vi "ReadScheduleFile.vi"(7 "Enum":enum16{"Load", "Get"}(ring), 8 "Team Info / Schedule File":path=path "C:/Program Files/FIRST LEGO LEAGUE TOURNAMENT/data/schedule.csv") -> (0 "error out":errorcluster, 1 "Table Stats":T1, 2 "PracticeMatches":string[][](array[string])=[["1", "1060", "3132", "5421", "77"], ["2", "510", "2128", "5441", "781"], ["3", "305", "98", "5470", "1951"], ["4", "685", "1429", "5481", "340"], ["5", "486", "3730", "5420", "12"], ["6", "1857", "3019", "5411", "390"], ["7", "5391", "1105", "5400", "2580"], ["8", "729", "2216", "5480", "822"], ["9", "752", "266", "5371", "3187"], ["10", "3622", "4861", "5360", "517"], ["11", "1633", "2882", "0", "0"], ["12", "3132", "5421", "77", "1060"], ["13", "2128", "5441", "781", "510"], ["14", "98", "5470", "1951", "305"], ["15", "1429", "5481", "340", "685"], ["16", "3730", "5420", "12", "486"], ["17", "3019", "5411", "390", "1857"], ["18", "1105", "5400", "2580", "5391"], ["19", "2216", "5480", "822", "729"], ["20", "266", "5371", "3187", "752"], ["21", "4861", "517", "5360", "1633"], ["22", "0", "0", "3622", "2882"], ["23", "74", "96", "5440", "3188"], ["24", "439", "13", "5410", "5471"], ["25", "3817", "2641", "5401", "1694"], ["26", "151", "5422", "5390", "647"], ["27", "1447", "420", "5370", "280"], ["28", "2880", "66", "5361", "3022"], ["29", "164", "22", "5351", "744"], ["30", "5423", "2708", "5432", "2469"], ["31", "4698", "995", "5430", "1"], ["32", "2961", "1707", "5353", "5315"], ["33", "13", "5471", "439", "5410"], ["34", "96", "3188", "74", "5440"], ["35", "5422", "647", "151", "5390"], ["36", "2641", "1694", "3817", "5401"], ["37", "66", "3022", "2880", "5361"], ["38", "420", "280", "1447", "5370"], ["39", "2708", "2469", "5423", "5432"], ["40", "22", "744", "164", "5351"], ["41", "1707", "5315", "2961", "5353"], ["42", "995", "1", "4698", "5430"]], 3 "RankingMatches":string[][](array[string])=[["1", "74", "96", "5440", "3188"], ["2", "439", "13", "5410", "5471"], ["3", "3817", "2641", "5401", "1694"], ["4", "151", "5422", "5390", "647"], ["5", "1447", "420", "5370", "280"], ["6", "2880", "66", "5361", "3022"], ["7", "164", "22", "5351", "744"], ["8", "5423", "2708", "5432", "2469"], ["9", "4698", "995", "5430", "1"], ["10", "2961", "1707", "5353", "5315"], ["11", "1060", "3132", "5421", "77"], ["12", "510", "2128", "5441", "781"], ["13", "305", "98", "5470", "1951"], ["14", "685", "1429", "5481", "340"], ["15", "486", "3730", "5420", "12"], ["16", "1857", "3019", "5411", "390"], ["17", "5391", "1105", "5400", "2580"], ["18", "729", "2216", "5480", "822"], ["19", "752", "266", "5371", "3187"], ["20", "3622", "4861", "5360", "517"], ["21", "1633", "2882", "0", "0"], ["22", "96", "3188", "74", "5440"], ["23", "13", "5471", "439", "5410"], ["24", "2641", "1694", "3817", "5401"], ["25", "5422", "647", "151", "5390"], ["26", "420", "280", "1447", "5370"], ["27", "66", "3022", "2880", "5361"], ["28", "22", "744", "164", "5351"], ["29", "2708", "2469", "5423", "5432"], ["30", "995", "1", "4698", "5430"], ["31", "1707", "5315", "2961", "5353"], ["32", "3132", "77", "1060", "5421"], ["33", "2128", "781", "510", "5441"], ["34", "98", "1951", "305", "5470"], ["35", "1429", "340", "685", "5481"], ["36", "3730", "12", "486", "5420"], ["37", "3019", "390", "1857", "5411"], ["38", "1105", "2580", "5391", "5400"], ["39", "2216", "822", "729", "5480"], ["40", "266", "3187", "752", "5371"], ["41", "4861", "517", "5360", "1633"], ["42", "0", "0", "3622", "2882"], ["43", "96", "5440", "3188", "74"], ["44", "13", "5410", "5471", "439"], ["45", "2641", "5401", "1694", "3817"], ["46", "5422", "5390", "647", "151"], ["47", "420", "5370", "280", "1447"], ["48", "66", "5361", "3022", "2880"], ["49", "22", "5351", "744", "164"], ["50", "2708", "5432", "2469", "5423"], ["51", "995", "5430", "1", "4698"], ["52", "1707", "5353", "5315", "2961"], ["53", "3132", "5421", "77", "1060"], ["54", "2128", "5441", "781", "510"], ["55", "98", "5470", "1951", "305"], ["56", "1429", "5481", "340", "685"], ["57", "3730", "5420", "12", "486"], ["58", "3019", "5411", "390", "1857"], ["59", "1105", "5400", "2580", "5391"], ["60", "2216", "5480", "822", "729"], ["61", "266", "5371", "3187", "752"], ["62", "5360", "2882", "4861", "1633"], ["63", "0", "0", "3622", "517"]], 4 "Table Names":string[](array[string]), 5 "Team Information":cluster{string, "[0]":string, "[1]":string}[](array[cluster])=[{"74, The Stonecutters", "[0]"="74", "[1]"="The Stonecutters"}, {"96, ROBOWhizards Rookies", "[0]"="96", "[1]"="ROBOWhizards Rookies"}, {"5440, Ambrose Argonauts", "[0]"="5440", "[1]"="Ambrose Argonauts"}, {"3188, RoboRays", "[0]"="3188", "[1]"="RoboRays"}, {"439, Vicious Vikings", "[0]"="439", "[1]"="Vicious Vikings"}, {"13, TechnoDudes", "[0]"="13", "[1]"="TechnoDudes"}, {"5410, The Rockys", "[0]"="5410", "[1]"="The Rockys"}, {"5471, ACATL", "[0]"="5471", "[1]"="ACATL"}, {"3817, Undersea United", "[0]"="3817", "[1]"="Undersea United"}, {"2641, FIRSTfruits", "[0]"="2641", "[1]"="FIRSTfruits"}, {"5401, Shuma", "[0]"="5401", "[1]"="Shuma"}, {"1694, S.P.I.D.E.R.S.", "[0]"="1694", "[1]"="S.P.I.D.E.R.S."}, {"151, Robot Masters", "[0]"="151", "[1]"="Robot Masters"}, {"5422, Vikings", "[0]"="5422", "[1]"="Vikings"}, {"5390, Robo Alliance", "[0]"="5390", "[1]"="Robo Alliance"}, {"647, Roboteers", "[0]"="647", "[1]"="Roboteers"}, {"1447, Long Island Robotics Club (LIRC)", "[0]"="1447", "[1]"="Long Island Robotics Club (LIRC)"}, {"420, Legos Inc.", "[0]"="420", "[1]"="Legos Inc."}, {"5370, SAP Eleven", "[0]"="5370", "[1]"="SAP Eleven"}, {"280, MindStorm Troopers", "[0]"="280", "[1]"="MindStorm Troopers"}, {"2880, Aquatic Ninjas", "[0]"="2880", "[1]"="Aquatic Ninjas"}, {"66, The Sea Monkeys", "[0]"="66", "[1]"="The Sea Monkeys"}, {"5361, China AAC", "[0]"="5361", "[1]"="China AAC"}, {"3022, Vikinetics", "[0]"="3022", "[1]"="Vikinetics"}, {"164, Beach Busters", "[0]"="164", "[1]"="Beach Busters"}, {"22, Aquatic Configurators", "[0]"="22", "[1]"="Aquatic Configurators"}, {"5351, EXPLOROBOTS", "[0]"="5351", "[1]"="EXPLOROBOTS"}, {"744, RCXRM  (Roberts Creek Xtreme Robotic Minds)", "[0]"="744", "[1]"="RCXRM  (Roberts Creek Xtreme Robotic Minds)"}, {"5423, RoboGenius", "[0]"="5423", "[1]"="RoboGenius"}, {"2708, Ferocious Furballs and Two Dudes", "[0]"="2708", "[1]"="Ferocious Furballs and Two Dudes"}, {"5432, SAPmarine Against Pollution", "[0]"="5432", "[1]"="SAPmarine Against Pollution"}, {"2469, Yellow Submarines", "[0]"="2469", "[1]"="Yellow Submarines"}, {"4698, TechnoGirls", "[0]"="4698", "[1]"="TechnoGirls"}, {"995, Oscarville Technobots", "[0]"="995", "[1]"="Oscarville Technobots"}, {"5430, Jet-Net (Hofstad College)", "[0]"="5430", "[1]"="Jet-Net (Hofstad College)"}, {"1, S.M.A.R.T", "[0]"="1", "[1]"="S.M.A.R.T"}, {"2961, Robotrics", "[0]"="2961", "[1]"="Robotrics"}, {"1707, RoboRockers", "[0]"="1707", "[1]"="RoboRockers"}, {"5353, Electric Eels", "[0]"="5353", "[1]"="Electric Eels"}, {"5315, St. Dominic Sea Dragons", "[0]"="5315", "[1]"="St. Dominic Sea Dragons"}, {"1060, RoboRage", "[0]"="1060", "[1]"="RoboRage"}, {"3132, JAMBots - Sandy Run Robotics Club", "[0]"="3132", "[1]"="JAMBots - Sandy Run Robotics Club"}, {"5421, KID", "[0]"="5421", "[1]"="KID"}, {"77, LegoDogs", "[0]"="77", "[1]"="LegoDogs"}, {"510, Robotik", "[0]"="510", "[1]"="Robotik"}, {"2128, BIG APPLE ", "[0]"="2128", "[1]"="BIG APPLE "}, {"5441, Hexbotics", "[0]"="5441", "[1]"="Hexbotics"}, {"781, The Life Preservers", "[0]"="781", "[1]"="The Life Preservers"}, {"305, Seaweed Wackers 3.0", "[0]"="305", "[1]"="Seaweed Wackers 3.0"}, {"98, Deep Sea Boulder Beasts", "[0]"="98", "[1]"="Deep Sea Boulder Beasts"}, {"5470, Los Bananines ", "[0]"="5470", "[1]"="Los Bananines "}, {"1951, Lego Bots", "[0]"="1951", "[1]"="Lego Bots"}, {"685, Mach 6", "[0]"="685", "[1]"="Mach 6"}, {"1429, Overdrivers", "[0]"="1429", "[1]"="Overdrivers"}, {"5481, APOGEU", "[0]"="5481", "[1]"="APOGEU"}, {"340, St Francis Crusaders", "[0]"="340", "[1]"="St Francis Crusaders"}, {"486, North Andover Legotrons", "[0]"="486", "[1]"="North Andover Legotrons"}, {"3730, Nuclear Sharks", "[0]"="3730", "[1]"="Nuclear Sharks"}, {"5420, Ocean 12", "[0]"="5420", "[1]"="Ocean 12"}, {"12, Red Tide", "[0]"="12", "[1]"="Red Tide"}, {"1857, Gears in Motion", "[0]"="1857", "[1]"="Gears in Motion"}, {"3019, Belfast LEGO Lions", "[0]"="3019", "[1]"="Belfast LEGO Lions"}, {"5411, SAP All Stars", "[0]"="5411", "[1]"="SAP All Stars"}, {"390, Mad Robotists", "[0]"="390", "[1]"="Mad Robotists"}, {"5391, Robo Acers", "[0]"="5391", "[1]"="Robo Acers"}, {"1105, BotZealots", "[0]"="1105", "[1]"="BotZealots"}, {"5400, Blue Shark", "[0]"="5400", "[1]"="Blue Shark"}, {"2580, The One That Got Away", "[0]"="2580", "[1]"="The One That Got Away"}, {"729, Extra Technology", "[0]"="729", "[1]"="Extra Technology"}, {"2216, Robomasters", "[0]"="2216", "[1]"="Robomasters"}, {"5480, FREE ACCESS - CUARA BRASIL", "[0]"="5480", "[1]"="FREE ACCESS - CUARA BRASIL"}, {"822, Global Gators", "[0]"="822", "[1]"="Global Gators"}, {"752, SCS Penguins", "[0]"="752", "[1]"="SCS Penguins"}, {"266, Central SpaceLab One", "[0]"="266", "[1]"="Central SpaceLab One"}, {"5371, SAP Edisons", "[0]"="5371", "[1]"="SAP Edisons"}, {"3187, Children of the Square Table", "[0]"="3187", "[1]"="Children of the Square Table"}, {"3622, Enviro Nodes", "[0]"="3622", "[1]"="Enviro Nodes"}, {"4861, Mariners", "[0]"="4861", "[1]"="Mariners"}, {"5360, China AAC", "[0]"="5360", "[1]"="China AAC"}, {"517, Robo Monkeys", "[0]"="517", "[1]"="Robo Monkeys"}, {"1633, BX Ryders", "[0]"="1633", "[1]"="BX Ryders"}, {"2882, Team Nemo", "[0]"="2882", "[1]"="Team Nemo"}])   [LabVIEW 2013]
uses:
  <vilib>/regexp/Match Regular Expression.xnode
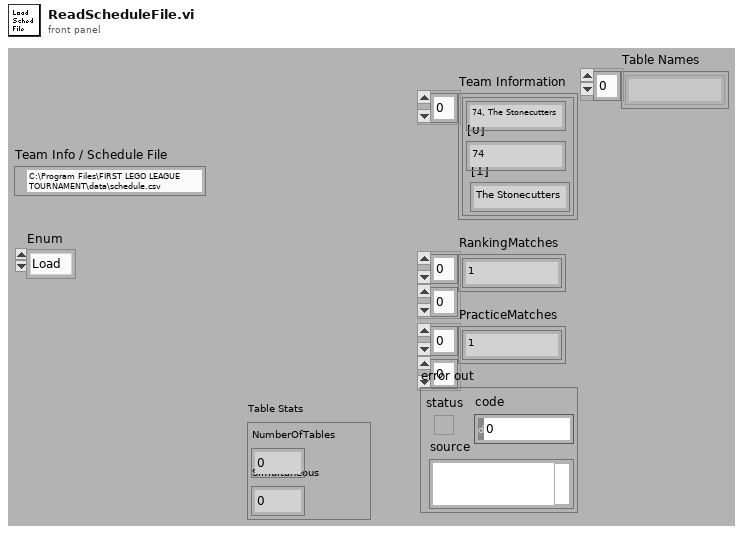
[diagram p1: front panel]
types:
  T1 = cluster{"NumberOfTables":i32, "Simultaneous":i32}
  T2 = cluster{"[0]":string, "[1]":string, "[2]":string, "[3]":string, "[4]":string, "[5]":string, "[6]":string, "[7]":string, "[8]":string}
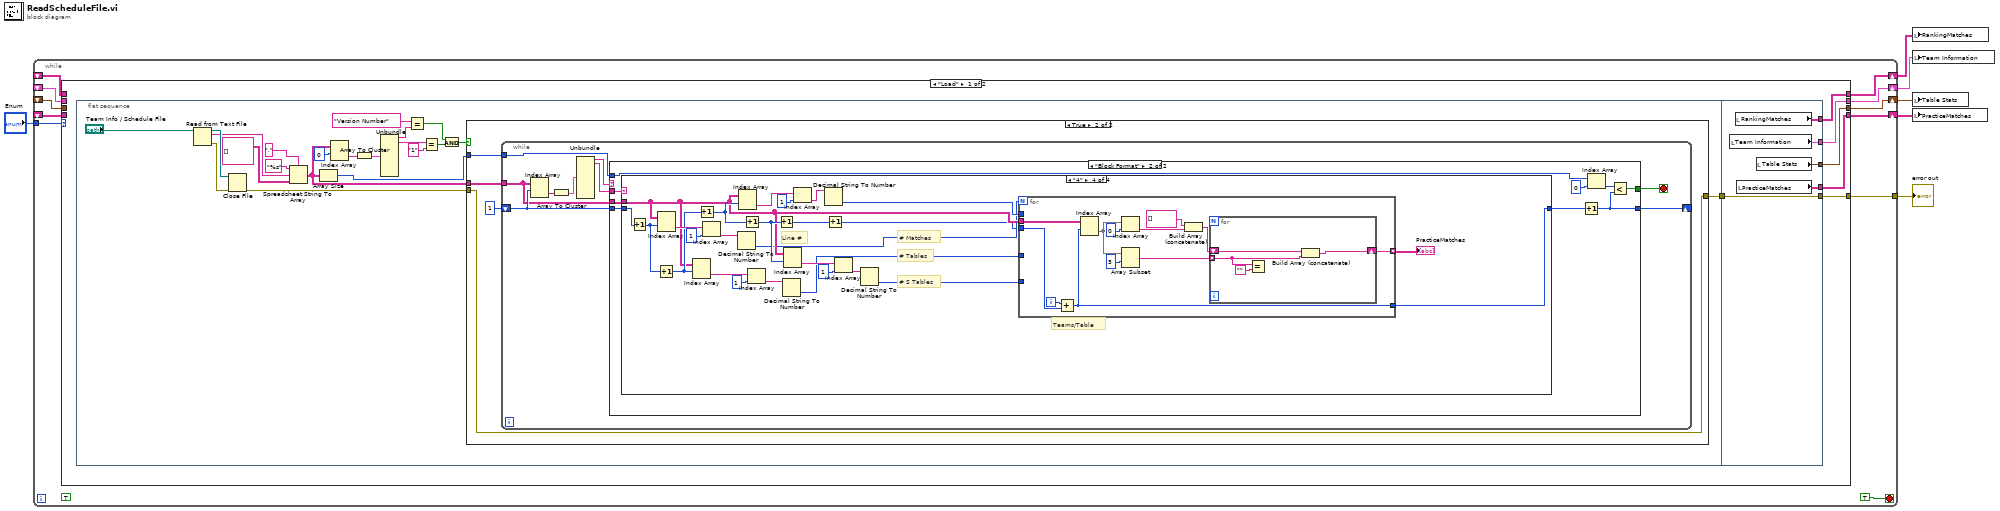
[diagram p0: block diagram]
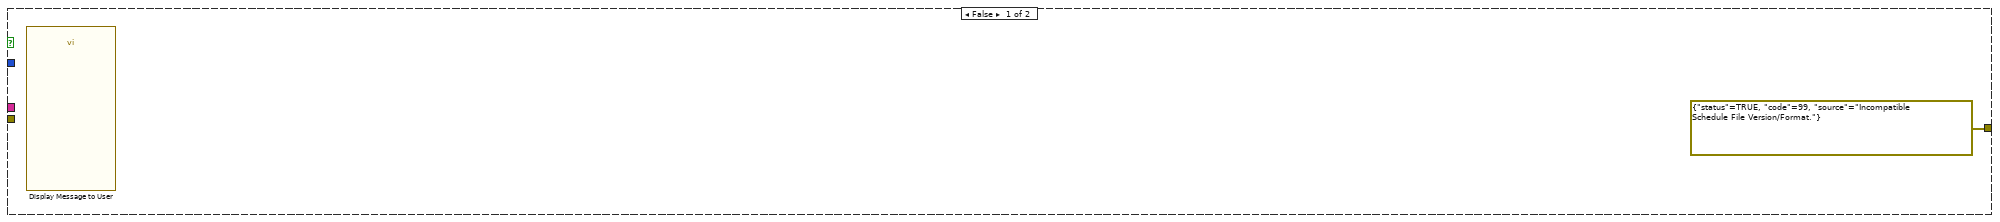
[diagram p2: hidden frame]
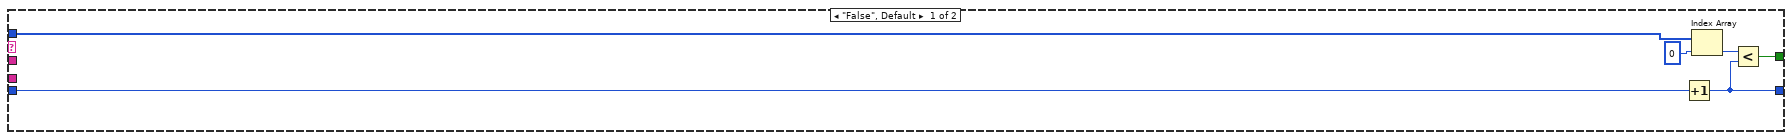
[diagram p3: hidden frame]
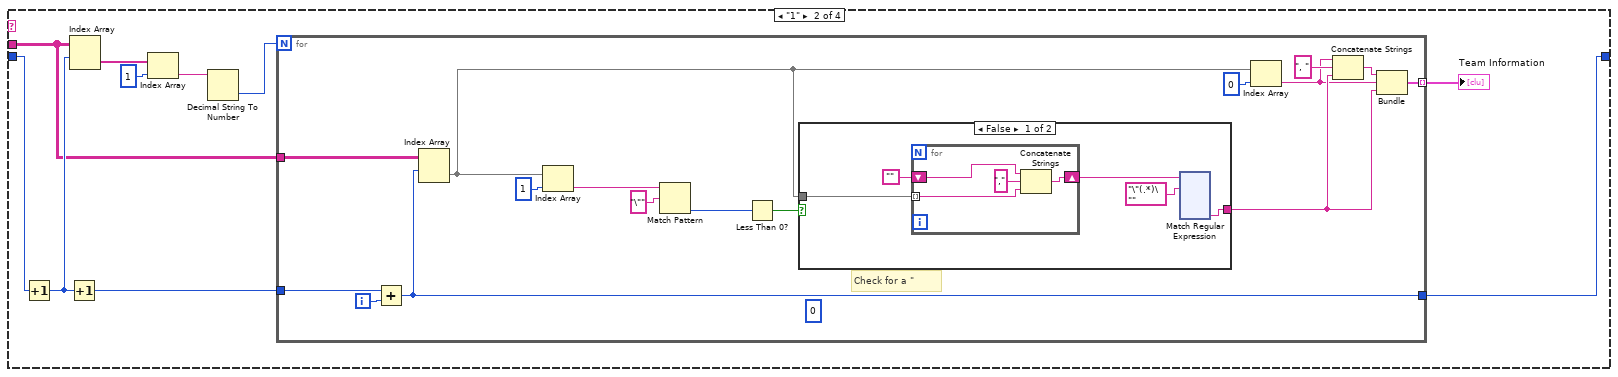
[diagram p5: hidden frame]
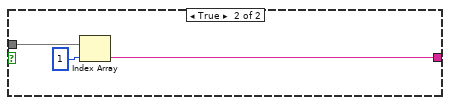
[diagram p6: hidden frame]
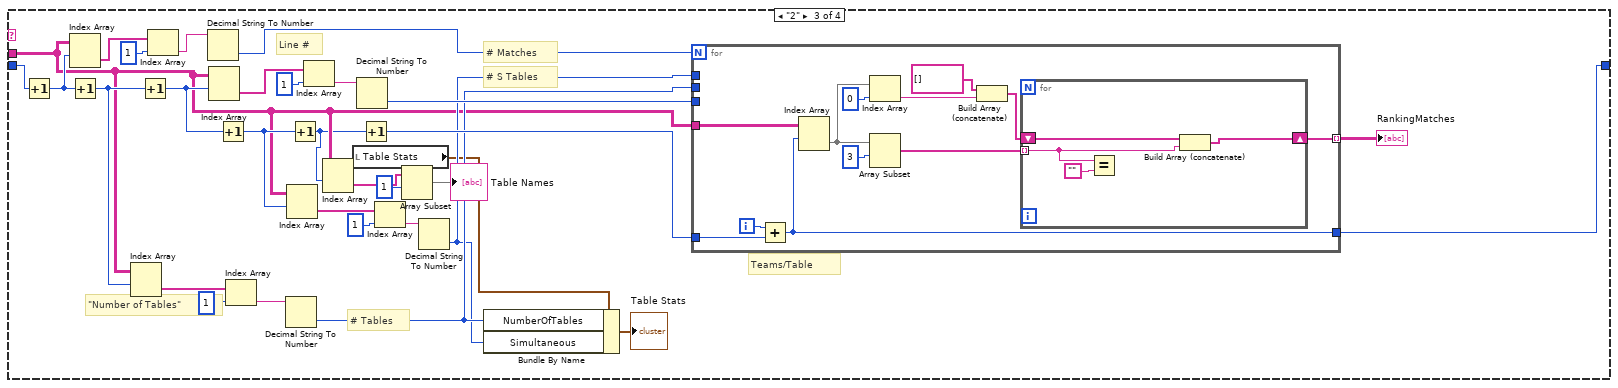
[diagram p7: hidden frame]
diagram:
  n1 = while {
    tunnel: [w17] -> w6
    shift-right: [w16] -> w4
    shift-left: _ -> [w10]
    shift-right: [w15] -> w3
    shift-left: _ -> [w9]
    shift-right: [w14] -> w2
    shift-left: _ -> [w8]
    shift-right: [w13] -> w1
    shift-left: _ -> [w7]
    tunnel: "Enum" -> [w11]
    stop <- TRUE stop-if-true
    (unwired) TRUE
    n2 = case shown="\"Load\"" w11 {
      tunnel: [w22 _] -> w17
      tunnel: [w18 w320] -> w16
      tunnel: [w21 w323] -> w15
      tunnel: [w20 w322] -> w14
      tunnel: [w19 w321] -> w13
      tunnel: w10 -> [_ w320]
      tunnel: w9 -> [_ w323]
      tunnel: w8 -> [_ w322]
      tunnel: w7 -> [_ w321]
      frame "Load" {
        n3 = flat-sequence {
          tunnel: [w25] -> w23
          tunnel: [w319] -> w22
          tunnel: w23 -> [w319]
          tunnel: [w318] -> w18
          tunnel: [w317] -> w21
          tunnel: [w315] -> w20
          tunnel: [w316] -> w19
          frame #0 {
            n4 = Read from Text File(file (use dialog)="Team Info / Schedule File") -> (refnum out=w40:refnum<file>, text=w39:string, error out=w41:errorcluster)  [unwired: 1 in, 3 out]
            n5 = Close File(refnum=w40, error in=w41) -> (error out=w26:errorcluster)  [unwired: 1 out]
            n6 = Spreadsheet String To Array(delimiter (Tab)=",", format string="%s", spreadsheet string=w39, array type (2D Dbl)=string[][] []) -> (array=w29:string[][])
            n7 = Array Size(array=w29) -> (size(s)=w28:i32[])
            n8 = Index Array(array=w29, index (row)=0) -> (element=w37:string[])  [unwired: 1 in]
            n9 = Array To Cluster(array=w37) -> (cluster=w36:T2)
            n10 = Unbundle(w36) -> ("[0]"=w30:string, "[1]"=w35:string)  [unwired: 7 out]
            n11 = Equal?(x="Version Number", y=w30) -> (x = y?=w32:bool)
            n12 = Equal?(x=w35, y="1") -> (x = y?=w33:bool)
            n13 = And(x=w32, y=w33) -> (x .and. y?=w27:bool)
            n14 = case shown="True" w27 {
              tunnel: w29 -> [_ w48]
              tunnel: w28 -> [_ w47]
              tunnel: w26 -> [_ w46]
              tunnel: [errorcluster {"status"=TRUE, "code"=99, "source"="Incompatible Schedule File Version/Format."} ("error out") w46] -> w25
              frame False {
                n15 = call "Display Message to User"() -> ()  [unwired: 3 in, 9 out]
              }
              frame True {
                n16 = while {
                  tunnel: w48 -> [w53]
                  shift-right: [w50] -> _
                  shift-left: 1 -> [w54]
                  tunnel: w47 -> [w52]
                  stop <- w51 stop-if-true
                  n17 = Index Array(array=w53, index (row)=w54) -> (element=w58:string[])  [unwired: 1 in]
                  n18 = Array To Cluster(array=w58) -> (cluster=w57:T2)
                  n19 = Unbundle(w57) -> ("[0]"=w56:string, "[1]"=w55:string)  [unwired: 7 out]
                  n20 = case shown="\"Block Format\"" w56 {
                    tunnel: w55 -> [_ w73]
                    tunnel: w54 -> [w64 w72]
                    tunnel: w53 -> [_ w71]
                    tunnel: w52 -> [w61 w68]
                    tunnel: [w59 w70] -> w51
                    tunnel: [w60 w65] -> w50
                    frame "False", Default {
                      n21 = Increment(x=w64) -> (x+1=w60:i32)
                      n22 = Index Array(array=w61, index=0) -> (element=w62:i32)
                      n23 = Less?(x=w62, y=w60) -> (x < y?=w59:bool)
                    }
                    frame "Block Format" {
                      n24 = case shown="\"4\"" w73 {
                        tunnel: w72 -> [w74 w84 w256 w298]
                        tunnel: w71 -> [_ w81 w230 w277]
                        tunnel: [w74 w80 w237 w275] -> w67
                        frame "False", Default {
                        }
                        frame "1" {
                          n25 = Increment(x=w84) -> (x+1=w83:i32)
                          n26 = Increment(x=w83) -> (x+1=w82:i32)
                          n27 = Index Array(array=w81, index (row)=w83) -> (element=w77:string[])  [unwired: 1 in]
                          n28 = Index Array(array=w77, index=1) -> (element=w78:string)
                          n29 = Decimal String To Number(string=w78) -> (number=w79:i32)  [unwired: 3 out]
                          n30 = for {
                            N: w79 -> [_]
                            tunnel: w82 -> [w99]
                            tunnel: w81 -> [w98]
                            tunnel: [w95] -> w75 mode=indexing
                            tunnel: [w94] -> w80
                            i -> [w100]
                            (unwired) 0
                            # "Check for a \""
                            n31 = Add(x=w99, y=w100) -> (x+y=w94:i32)
                            n32 = Index Array(array=w98, index (row)=w94) -> (element=w87:string[])  [unwired: 1 in]
                            n33 = Index Array(array=w87, index=1) -> (element=w88:string)
                            n34 = Match Pattern(string=w88, regular expression="\"") -> (offset past match=w85:i32)  [unwired: 4 out]
                            n35 = Less Than 0?(x=w85) -> (x < 0?=w86:bool)
                            n36 = case shown="False" w86 {
                              tunnel: [w102 w223] -> w93
                              tunnel: w87 -> [w101 w224]
                              frame False {
                                n37 = for {
                                tunnel: w101 -> [w220] mode=indexing
                                shift-right: [w219] -> w103
                                shift-left: "" -> [w222]
                                n38 = Concatenate Strings(w222, "," ("string"), w220) -> (w219:string)
                                }
                                n39 = xnode "Match Regular Expression"("input string"=w103, "regular expression"="\"(.*)\"") -> ("submatch 1"=w102:string)  [unwired: 2 in, 7 out]
                              }
                              frame True {
                                n40 = Index Array(array=w224, index=1) -> (element=w223:string)
                              }
                            }
                            n41 = Index Array(array=w87, index=0 ("index (row)")) -> (element=w91:string)
                            n42 = Concatenate Strings(w91, ", " ("string"), w93) -> (w97:string)
                            n43 = Bundle(w97, w91, "submatch 1"=w93) -> (w95:cluster{string, string, "submatch 1":string})  [unwired: 1 out]
                          }
                          "Team Information" <- w75
                        }
                        frame "2" {
                          # "\"Number of Tables\""
                          # "# S Tables"
                          # "Teams/Table"
                          # "# Tables"
                          # "Line #"
                          # "# Matches"
                          n44 = Increment(x=w256) -> (x+1=w252:i32)
                          n45 = Index Array(array=w230, index (row)=w252) -> (element=w254:string[])  [unwired: 1 in]
                          n46 = Increment(x=w252) -> (x+1=w245:i32)
                          n47 = Index Array(array=w230, index (row)=w245) -> (element=w250:string[])  [unwired: 1 in]
                          n48 = Increment(x=w245) -> (x+1=w241:i32)
                          n49 = Index Array(array=w254, index=1) -> (element=w255:string)
                          n50 = Decimal String To Number(string=w255) -> (number=w238:i32)  [unwired: 3 out]
                          n51 = Index Array(array=w230, index (row)=w241) -> (element=w247:string[])  [unwired: 1 in]
                          n52 = Increment(x=w241) -> (x+1=w240:i32)
                          n53 = Index Array(array=w250, index=1) -> (element=w249:string)
                          n54 = Decimal String To Number(string=w249) -> (number=w235:i32)  [unwired: 3 out]
                          n55 = Index Array(array=w230, index (row)=w240) -> (element=w243:string[])  [unwired: 1 in]
                          n56 = Increment(x=w240) -> (x+1=w229:i32)
                          n57 = Index Array(array=w247, index=1) -> (element=w248:string)
                          n58 = Index Array(array=w230, index (row)=w229) -> (element=w228:string[])  [unwired: 1 in]
                          n59 = local read "Table Stats"() -> (w231:T1)
                          n60 = Decimal String To Number(string=w248) -> (number=w239:i32)  [unwired: 3 out]
                          n61 = Increment(x=w229) -> (x+1=w236:i32)
                          n62 = Index Array(array=w243, index=1) -> (element=w242:string)
                          n63 = Array Subset(array=w228, index=1) -> (→"Table Names":string[])  [unwired: 1 in]
                          n64 = Decimal String To Number(string=w242) -> (number=w234:i32)  [unwired: 3 out]
                          n65 = Bundle By Name(cluster=w231, "NumberOfTables"=w235, "Simultaneous"=w234) -> (→"Table Stats":T1)
                          n66 = for {
                            N: w238 -> [_]
                            tunnel: w230 -> [w266]
                            tunnel: w235 -> [_]
                            tunnel: w239 -> [_]
                            tunnel: w234 -> [_]
                            tunnel: w236 -> [w267]
                            tunnel: [w261] -> w232 mode=indexing
                            tunnel: [w257] -> w237
                            i -> [w268]
                            n67 = Add(x=w268, y=w267) -> (x+y=w257:i32)
                            n68 = Index Array(array=w266, index (row)=w257) -> (element=w264:string[])  [unwired: 1 in]
                            n69 = Index Array(array=w264, index=0) -> (element=w259:string)
                            n70 = Array Subset(array=w264, index=3) -> (w262:string[])  [unwired: 1 in]
                            n71 = Build Array (concatenate)(string[] [], w259) -> (w260:string[])
                            n72 = for {
                              shift-right: [w269] -> w261
                              shift-left: w260 -> [w270]
                              tunnel: w262 -> [w271] mode=indexing
                              n73 = Equal?(x=w271, y="") -> ()  [unwired: 1 out]
                              n74 = Build Array (concatenate)(w270, w271) -> (w269:string[])
                            }
                          }
                          "RankingMatches" <- w232
                        }
                        frame "4" {
                          # "# S Tables"
                          # "Teams/Table"
                          # "# Tables"
                          # "Line #"
                          # "# Matches"
                          n75 = Increment(x=w298) -> (x+1=w294:i32)
                          n76 = Index Array(array=w277, index (row)=w294) -> (element=w296:string[])  [unwired: 1 in]
                          n77 = Increment(x=w294) -> (x+1=w287:i32)
                          n78 = Index Array(array=w277, index (row)=w287) -> (element=w292:string[])  [unwired: 1 in]
                          n79 = Increment(x=w287) -> (x+1=w283:i32)
                          n80 = Index Array(array=w296, index=1) -> (element=w297:string)
                          n81 = Decimal String To Number(string=w297) -> (number=w276:i32)  [unwired: 3 out]
                          n82 = Index Array(array=w277, index (row)=w283) -> (element=w289:string[])  [unwired: 1 in]
                          n83 = Increment(x=w283) -> (x+1=w282:i32)
                          n84 = Index Array(array=w292, index=1) -> (element=w291:string)
                          n85 = Increment(x=w282) -> (x+1=w278:i32)
                          n86 = Decimal String To Number(string=w291) -> (number=w279:i32)  [unwired: 3 out]
                          n87 = Index Array(array=w277, index (row)=w282) -> (element=w285:string[])  [unwired: 1 in]
                          n88 = Index Array(array=w289, index=1) -> (element=w290:string)
                          n89 = Decimal String To Number(string=w290) -> (number=w280:i32)  [unwired: 3 out]
                          n90 = Increment(x=w278) -> (x+1=w274:i32)
                          n91 = Index Array(array=w285, index=1) -> (element=w284:string)
                          n92 = Decimal String To Number(string=w284) -> (number=w281:i32)  [unwired: 3 out]
                          n93 = for {
                            N: w276 -> [_]
                            tunnel: w277 -> [w308]
                            tunnel: w279 -> [_]
                            tunnel: w280 -> [_]
                            tunnel: w281 -> [_]
                            tunnel: w274 -> [w309]
                            tunnel: [w303] -> w273 mode=indexing
                            tunnel: [w299] -> w275
                            i -> [w310]
                            n94 = Add(x=w310, y=w309) -> (x+y=w299:i32)
                            n95 = Index Array(array=w308, index (row)=w299) -> (element=w306:string[])  [unwired: 1 in]
                            n96 = Index Array(array=w306, index=0) -> (element=w301:string)
                            n97 = Array Subset(array=w306, index=3) -> (w304:string[])  [unwired: 1 in]
                            n98 = Build Array (concatenate)(string[] [], w301) -> (w302:string[])
                            n99 = for {
                              shift-right: [w311] -> w303
                              shift-left: w302 -> [w312]
                              tunnel: w304 -> [w313] mode=indexing
                              n100 = Equal?(x=w313, y="") -> ()  [unwired: 1 out]
                              n101 = Build Array (concatenate)(w312, w313) -> (w311:string[])
                            }
                          }
                          "PracticeMatches" <- w273
                        }
                      }
                      n102 = Increment(x=w67) -> (x+1=w65:i32)
                      n103 = Index Array(array=w68, index=0) -> (element=w66:i32)
                      n104 = Less?(x=w66, y=w65) -> (x < y?=w70:bool)
                    }
                  }
                }
              }
            }
          }
          frame #1 {
            n105 = local read "Team Information"() -> (w317:cluster{string, "[0]":string, "[1]":string}[])
            n106 = local read "RankingMatches"() -> (w318:string[][])
            n107 = local read "PracticeMatches"() -> (w316:string[][])
            n108 = local read "Table Stats"() -> (w315:T1)
          }
        }
      }
      frame "Get", Default {
      }
    }
  }
  "error out" <- w6
  n109 = local write "RankingMatches"(w4) -> ()
  n110 = local write "Team Information"(w3) -> ()
  n111 = local write "Table Stats"(w2) -> ()
  n112 = local write "PracticeMatches"(w1) -> ()
